vi "Bearing-Heading Converter.vi"(8 "error in (no error)":errorcluster, 9 "Bearing in":dbl, 10 "Heading in":i32, 11 "Simulator in":refnum<class "Simulator.lvclass">) -> (0 "error out":errorcluster, 1 "Heading out":i32, 2 "Bearing out":dbl, 3 "Simulator out":refnum<class "Simulator.lvclass">)   [LabVIEW 2011, in "Simulator.lvclass"]
uses:
  Simulator.lvclass
  Simulator.lvclass/Simulator.ctl
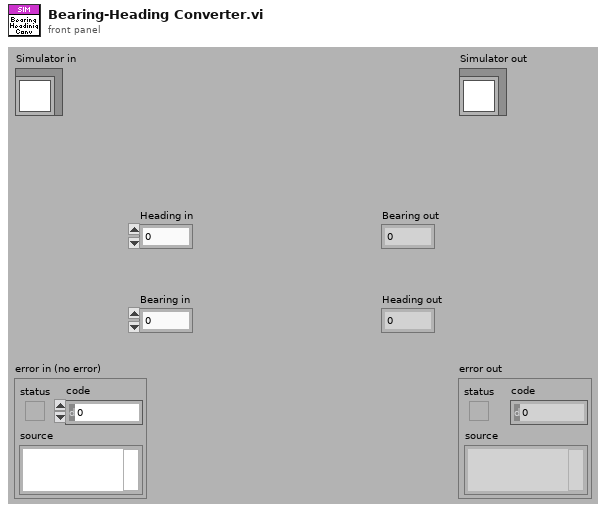
[diagram p1: front panel]
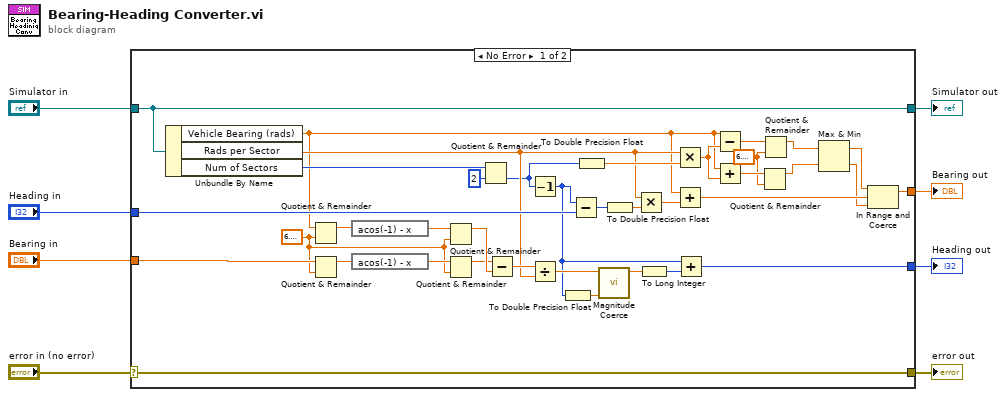
[diagram p0: block diagram]
diagram:
  n1 = case shown="No Error" "error in (no error)" {
    selector: "error in (no error)" -> [w45 w49]
    tunnel: [w45 w49] -> w7
    tunnel: [w44 w48] -> w5
    tunnel: "Simulator in" -> [w44 w48]
    tunnel: "Heading in" -> [w41 w47]
    tunnel: [w37 w46] -> w3
    tunnel: "Bearing in" -> [w26 w46]
    tunnel: [w22 w47] -> w1
    frame No Error {
      w13 = 6.283185307179586
      w27 = 6.283185307179586
      n2 = Unbundle By Name(w44) -> ("Vehicle Bearing (rads)"=w20:dbl, "Rads per Sector"=w24:dbl, "Num of Sectors"=w43:i32)
      n3 = Quotient & Remainder(x=w20, y=w13) -> (x-y*floor(x/y)=w19:dbl)  [unwired: 1 out]
      n4 = Quotient & Remainder(x=w26, y=w13) -> (x-y*floor(x/y)=w18:dbl)  [unwired: 1 out]
      n5 = expression code="acos(-1) - x"(w19) -> (w17:dbl)
      n6 = expression code="acos(-1) - x"(w18) -> (w16:dbl)
      n7 = Quotient & Remainder(x=w17, y=w13) -> (x-y*floor(x/y)=w15:dbl)  [unwired: 1 out]
      n8 = Quotient & Remainder(x=w16, y=w13) -> (x-y*floor(x/y)=w14:dbl)  [unwired: 1 out]
      n9 = Quotient & Remainder(x=w43, y=2) -> (floor(x/y)=w21:i32)  [unwired: 1 out]
      n10 = Subtract(x=w14, y=w15) -> (x-y=w25:dbl)
      n11 = Decrement(x=w21) -> (x-1=w9:i32)
      n12 = Divide(x=w25, y=w24) -> (x/y=w12:dbl)
      n13 = To Double Precision Float(number=w9) -> (double precision float=w10:dbl)
      n14 = Subtract(x=w9, y=w41) -> (x-y=w40:i32)
      n15 = To Double Precision Float(number=w21) -> (double precision float=w36:dbl)
      n16 = call "Magnitude Coerce.vi"("Magnitude Limit"=w10, "x"=w12) -> ("Coerce(x)"=w11:dbl)  [unwired: 8 in, 1 out]
      n17 = To Double Precision Float(number=w40) -> (double precision float=w39:dbl)
      n18 = Multiply(x=w24, y=w39) -> (x*y=w38:dbl)
      n19 = To Long Integer(number=w11) -> (32bit integer=w23:i32)
      n20 = Multiply(x=w24, y=w36) -> (x*y=w35:dbl)
      n21 = Add(x=w20, y=w38) -> (x+y=w34:dbl)
      n22 = Add(x=w9, y=w23) -> (x+y=w22:i32)
      n23 = Subtract(x=w20, y=w35) -> (x-y=w31:dbl)
      n24 = Add(x=w20, y=w35) -> (x+y=w29:dbl)
      n25 = Quotient & Remainder(x=w29, y=w27) -> (x-y*floor(x/y)=w28:dbl)  [unwired: 1 out]
      n26 = Quotient & Remainder(x=w31, y=w27) -> (x-y*floor(x/y)=w30:dbl)  [unwired: 1 out]
      n27 = Max & Min(x=w30, y=w28) -> (max(x,y)=w33:dbl, min(x,y)=w32:dbl)
      n28 = In Range and Coerce(upper limit=w33, x=w34, lower limit=w32) -> (coerced(x)=w37:dbl)  [unwired: 1 out]
    }
    frame Error {
    }
  }
  "error out" <- w7
  "Simulator out" <- w5
  "Bearing out" <- w3
  "Heading out" <- w1
